vi "BangBang_Execute.vi"(9 "Setpoint":dbl, 10 "Measurment":dbl, 11 "Tolerance":dbl) -> (1 "AtSetpoint":bool, 3 "ControlOutput":dbl, 4 "out BANG_BANG":T1 {"Measurment" format="%13.5p"; "Setpoint" format="%13.5p"; "Tolerance" format="%13.5p"})   [LabVIEW 2019, in "Trajectory_Library.lvlib"]
doc: "Implements and executes bang-bang controller, which outputs either 0 or 1 depending on whether the measurement is less than the setpoint. This maximally-aggressive control approach works very well for velocity control of high-inertia mechanisms, and poorly on most other things. \n \nNote that this is an *asymmetric* bang-bang controller - it will not exert any control effort in the reverse direction (e.g. it won't try to slow down an over-speeding shooter wheel). This asymmetry is *extremely important.* Bang-bang control is extremely simple, but also potentially hazardous. Always ensure that your motor controllers are set to \"coast\" before attempting to\ncontrol them with a bang-bang controller.\n\nAlways ensure that your motor controllers are set to \"coast\" before attempting to control\nthem with a bang-bang controller.\n\nInputs:\n - Tolerance -- Tolerance for \"at setpoint\"\n - measurement -- The most recent measurement of the process variable.\n - setpoint -- The setpoint for the process variable.\n\nOutputs:\n - ControlOutput -- The calculated motor output (0 or 1).\n - AtSetpoint -- Returns TRUE if within error tolerance. \n - BangBang -- Data clusterReturns the calculated control output."
uses:
  BANG_BANG.ctl
  Trajectory_Library.lvlib
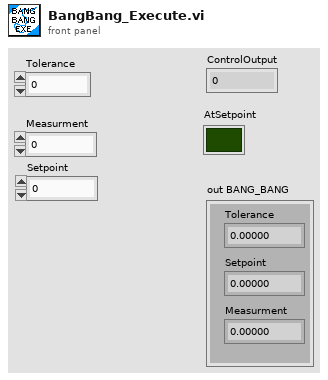
[diagram p1: front panel]
types:
  T1 = typedef "Trajectory_Library.lvlib/BANG_BANG.ctl" = cluster{"Tolerance":dbl, "Setpoint":dbl, "Measurment":dbl}
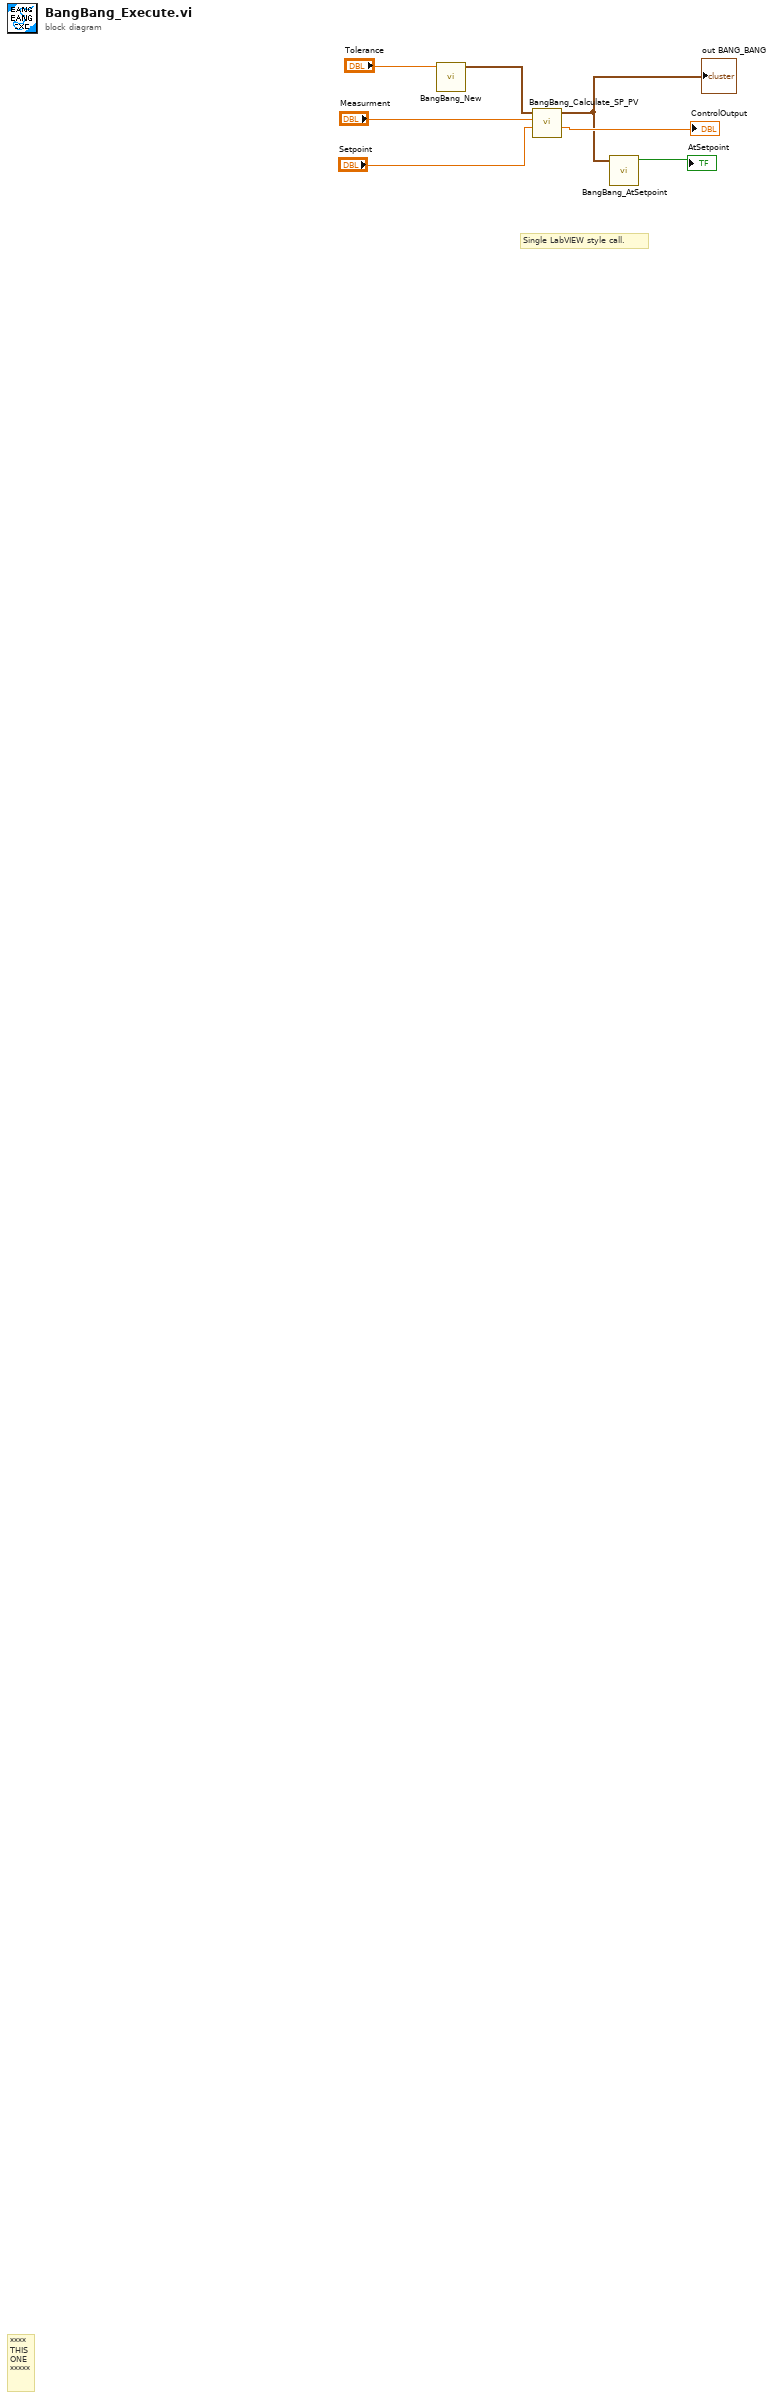
[diagram p0: block diagram]
diagram:
  # "Single LabVIEW style call."
  # "****\nTHIS\nONE\n*****"
  n1 = call "BangBang_New.vi"("Tolerance"="Tolerance") -> ("BANG_BANG"=w6:T1)  [unwired: 10 in]
  n2 = call "BangBang_Calculate_SP_PV.vi"("Setpoint"="Setpoint", "Measurment"="Measurment", "BANG_BANG"=w6) -> ("ControlOutput"=→"ControlOutput":dbl, "out BANG_BANG"=w1:T1)  [unwired: 7 in]
  "out BANG_BANG" <- w1
  n3 = call "BangBang_AtSetpoint.vi"("BANG_BANG"=w1) -> ("AtSetpoint"=→"AtSetpoint":bool)  [unwired: 10 in]
